vi "Commutator_query_CMD.vi"(9 "CMD":string="*IDN?", 11 "VISA in":T1) -> (0 "Err text":string, 1 "Err no":i16, 2 "RX error":bool, 3 "VISA out":T1, 4 "Response":string)   [LabVIEW 2011]
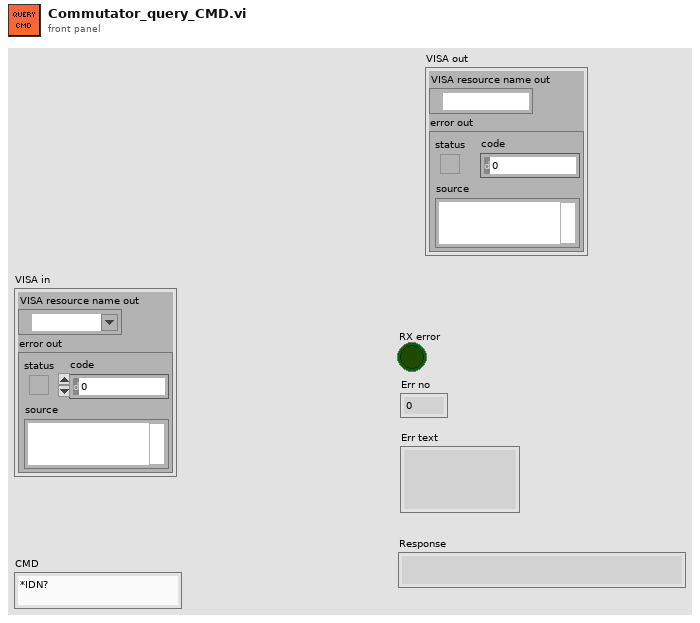
[diagram p1: front panel]
types:
  T1 = cluster{"VISA resource name out":refnum<visa-resource-name>, "error out":errorcluster}
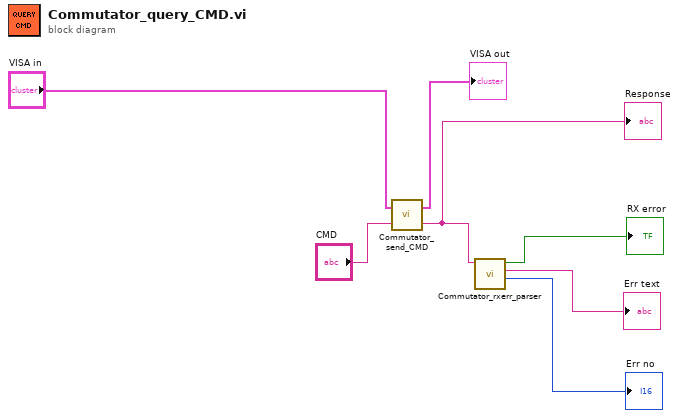
[diagram p0: block diagram]
diagram:
  n1 = call "Commutator_send_CMD.vi"("CMD"="CMD", "VISA in"="VISA in") -> ("Response"=w6:string, "VISA out"=→"VISA out":T1)
  "Response" <- w6
  n2 = call "Commutator_rxerr_parser.vi"("String"=w6) -> ("Err no"=→"Err no":i16, "Err text"=→"Err text":string, "RX error"=→"RX error":bool)  [unwired: 8 in]
